vi "Create.vi"(8 "error in (no error)":errorcluster, 10 "Channel":u8=1 min=1 max=4, 11 "ILC DAC Factory in":refnum<class "ILC DAC Factory.lvclass">) -> (0 "error out":errorcluster, 2 "ILC DAC":refnum<class "ILC DAC.lvclass">, 3 "ILC DAC Factory out":refnum<class "ILC DAC Factory.lvclass">)   [LabVIEW 2015, in "ILC DAC Factory.lvclass"]
uses:
  ILC DAC Factory.lvclass
  ILC DAC/ILC DAC.lvclass
  ILC DAC 1/ILC DAC 1.lvclass
  ILC DAC 2/ILC DAC 2.lvclass
  ILC DAC 3/ILC DAC 3.lvclass
  ILC DAC 4/ILC DAC 4.lvclass
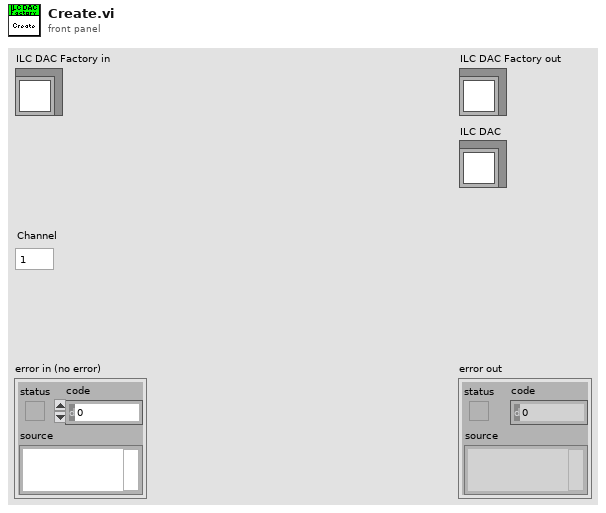
[diagram p1: front panel]
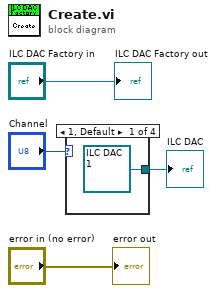
[diagram p0: block diagram]
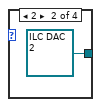
[diagram p2: hidden frame]
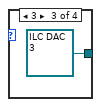
[diagram p3: hidden frame]
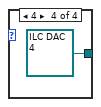
[diagram p4: hidden frame]
diagram:
  n1 = case shown="1, Default" "Channel" {
    tunnel: [refnum<class "ILC DAC 1.lvclass"> refnum ("ILCDAC1.lvclass") refnum<class "ILC DAC 2.lvclass"> refnum ("ILCDAC2.lvclass") refnum<class "ILC DAC 3.lvclass"> refnum ("ILCDAC3.lvclass") refnum<class "ILC DAC 4.lvclass"> refnum ("ILCDAC4.lvclass")] -> w1
    frame 1, Default {
    }
    frame 2 {
    }
    frame 3 {
    }
    frame 4 {
    }
  }
  "ILC DAC" <- w1
  "error out" <- "error in (no error)"
  "ILC DAC Factory out" <- "ILC DAC Factory in"
